vi "PCO_GetBatteryStatus.vi"(0 "ph":u64, 11 "error in (no error)":errorcluster {"code" format="%x"}) -> (3 "wBatteryLevel":u16, 4 "ph out":u64, 6 "ErrorMessage":i32 format="%x", 10 "wBatteryType":u16(ring) items=["no battery mounted"=0, "nickel metal hybrid type"=1, "lithium ion type"=2, "lithium iron phosphate type"=3, "battery dimax cs"=4, "unknown battery type"=65535], 12 "batteryIsCharged":bool, 13 "batteryMountedAndDetected":bool, 14 "powerSupplyAvailable":bool, 15 "error out":errorcluster {"code" format="%x"})   [LabVIEW 2019, in "SDK.lvlib" / "SpecialCommandsDimax.lvlib"]
doc: "<b>Description:</b>\nThis function returns the current state of the battery package connected to the camera.\n\n<b>Supported camera type:</b>\npco.dimax\n\n<b>Descriptor dependency:</b>\nwPowerDownModeDESC"
uses:
  SpecialCommandsDimax.lvlib
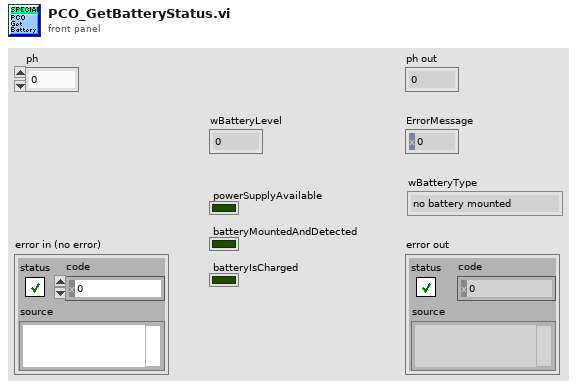
[diagram p1: front panel]
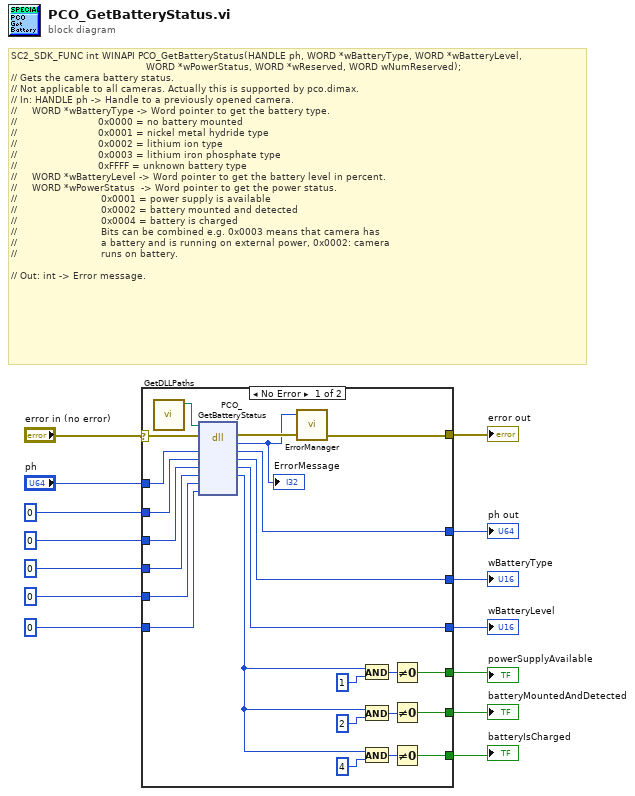
[diagram p0: block diagram]
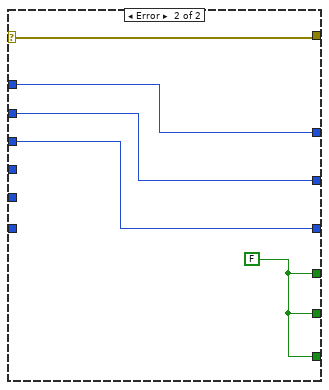
[diagram p2: hidden frame]
diagram:
  # "SC2_SDK_FUNC int WINAPI PCO_GetBatteryStatus(HANDLE ph, WORD *wBatteryType, WORD *wBatteryLevel,\n                                             WORD *wPowerStatus, WORD *wReserved, WORD wNumReserved);\n// Gets the camera battery status.\n// Not applicable to all cameras. Actually this is supported by pco.dimax.\n// In: HANDLE ph -> Handle to a previously opened camera.\n//     WORD *wBatteryType -> Word pointer to get the battery type.\n//                           0x0000 = no battery mounted\n//                           0x0001 = nickel metal hydride type\n//                           0x0002 = lithium ion type\n//                           0x0003 = lithium iron phosphate type\n//                           0xFFFF = unknown battery type\n//     WORD *wBatteryLevel -> Word pointer to get the battery level in percent.\n//     WORD *wPowerStatus  -> Word pointer to get the power status.\n//                            0x0001 = power supply is available\n//                            0x0002 = battery mounted and detected\n//                            0x0004 = battery is charged\n//                            Bits can be combined e.g. 0x0003 means that camera has\n//                            a battery and is running on external power, 0x0002: camera\n//                            runs on battery.\n\n// Out: int -> Error message."
  n1 = case shown="No Error" "error in (no error)" {
    selector: "error in (no error)" -> [w29 w43]
    tunnel: "ph" -> [w38 w42]
    tunnel: [w37 w42] -> w13
    tunnel: u16 0 ("wBatteryType") -> [w36 w41]
    tunnel: [w35 w41] -> w11
    tunnel: u16 0 ("wBatteryLevel") -> [w34 w40]
    tunnel: [w33 w40] -> w9
    tunnel: u16 0 ("wPowerStatus") -> [w32 _]
    tunnel: u16 0 ("wReserved") -> [w31 _]
    tunnel: [w27 w43] -> w6
    tunnel: u16 0 ("wReserved") -> [w30 _]
    tunnel: [w18 w39] -> w3
    tunnel: [w17 w39] -> w2
    tunnel: [w16 w39] -> w1
    frame No Error {
      n2 = call "GetDLLPaths.vi"() -> ("SC2_Cam_Path"=w15:path)  [unwired: 9 in, 2 out]
      n3 = dll-call lib="?" fn="PCO_GetBatteryStatus"(path in=w15, error in=w29, "ph"=w38, "wBatteryType"=w36, "wBatteryLevel"=w34, "wPowerStatus"=w32, "wReserved"=w31, "wNumReserved"=w30) -> (error out=w28:errorcluster, "return type"=w26:i32, "ph"=w37:u64, "wBatteryType"=w35:u16, "wBatteryLevel"=w33:u16, "wPowerStatus"=w25:u16)  [unwired: 3 in, 1 out]
      "ErrorMessage" <- w26
      n4 = call "ErrorManager.vi"("error in (no error)"=w28, "error code"=w26) -> ("error out"=w27:errorcluster)  [unwired: 3 in]
      n5 = And(x=w25, y=u16 1) -> (x .and. y?=w21:u16)
      n6 = And(x=w25, y=u16 2) -> (x .and. y?=w20:u16)
      n7 = And(x=w25, y=u16 4) -> (x .and. y?=w19:u16)
      n8 = Not Equal To 0?(x=w21) -> (x != 0?=w18:bool)
      n9 = Not Equal To 0?(x=w20) -> (x != 0?=w17:bool)
      n10 = Not Equal To 0?(x=w19) -> (x != 0?=w16:bool)
    }
    frame Error {
      w39 = FALSE
    }
  }
  "ph out" <- w13
  "wBatteryType" <- w11
  "wBatteryLevel" <- w9
  "powerSupplyAvailable" <- w3
  "error out" <- w6
  "batteryMountedAndDetected" <- w2
  "batteryIsCharged" <- w1
